vi "Config FGV - Set Current Project Item.vi"(11 "Set Current Project Item":string) -> ()   [LabVIEW 2014, in "i3-docs.lvlib"]
uses:
  i3-docs.lvlib
  Controls/config_fgv_actions.ctl
  Controls/config.ctl
  Controls/current_config.ctl
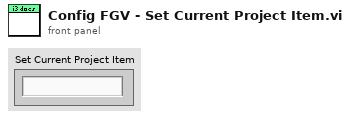
[diagram p1: front panel]
types:
  T1 = typedef "i3-docs.lvlib/config.ctl" = cluster{"Current Project":i32, "Project Configurations":T2[], "Current Project Item":string, "Finished?":bool, "Total Project Items":i32}
  T2 = typedef "i3-docs.lvlib/current_config.ctl" = cluster{"project file":path, "output directory":path}
  T3 = typedef "i3-docs.lvlib/config_fgv_actions.ctl" = enum16{"Initialize", "Set Current Project", "Get Current Config", "Set Current Project Item", "Finished"}
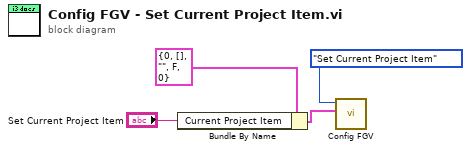
[diagram p0: block diagram]
diagram:
  n1 = Bundle By Name(cluster=T1 {"Current Project"=0, "Project Configurations"=[], "Current Project Item"="", "Finished?"=FALSE, "Total Project Items"=0} ("Application Configuration Input Helper"), "Current Project Item"="Set Current Project Item") -> (w2:T1)
  n2 = call "Config FGV.vi"("Application Configuration Input Helper"=w2, "Action"=config_fgv_actions."Set Current Project Item") -> ()  [unwired: 7 in, 3 out]
